vi "Destroy.vi"(8 "error in (no error)":errorcluster, 11 "SolarSystems M266 in":refnum<class "SolarSystems M266.lvclass">) -> (3 "SolarSystems M266 out":refnum<class "SolarSystems M266.lvclass">)   [LabVIEW 2014, in "SolarSystems M266.lvclass"]
uses:
  SolarSystems M266.lvclass
  Framework/Hardware/ParameterDevice/ParameterDevice.lvclass
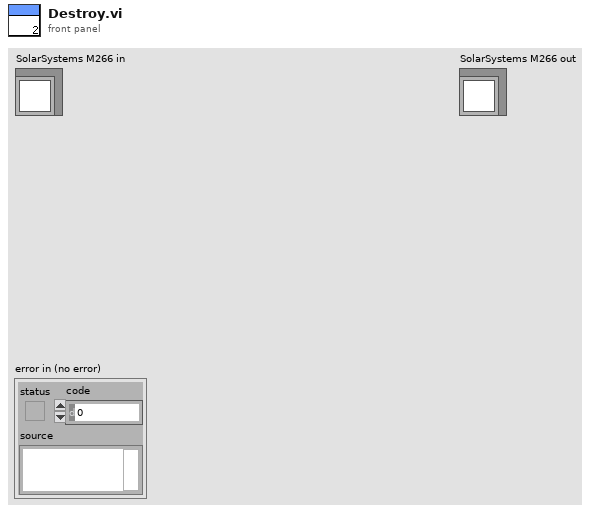
[diagram p1: front panel]
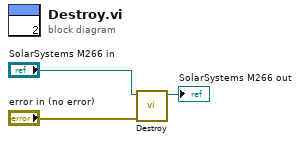
[diagram p0: block diagram]
diagram:
  n1 = call-parent "Destroy.vi"("error in (no error)"="error in (no error)", "Device in"="SolarSystems M266 in") -> ("Device out"=→"SolarSystems M266 out":refnum<class "SolarSystems M266.lvclass">)  [unwired: 9 in]
